vi "niFpgaSctlEmulationConstants.vi"() -> ()   [LabVIEW 2017]
panel:
  in  "MaxNumberOfLoops":i32=128
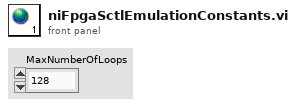
[diagram p1: front panel]
diagram:
